vi "Follow Path Speed Control.vi"(0 "Drivetrain":T11={"DevStatus"={"status"=FALSE, "code"=0, "source"=""}, "Motors[]"=[{"DeviceStatus"={"status"=FALSE, "code"=0, "source"=""}, "Type"=enum."PWM", "PWM"={"PWM Channel"=enum."PWM 1", "DeadBand"={"Name"="SPARK", "maxPositivePwm"=1500, "minPositivePwm"=1010, "centerPwm"=1005, "maxNegativePwm"=1000, "minNegativePwm"=500, "angularRange"=0}}, "CAN"={"Device Number"=0, "SetOutput VI Ref"=variant(refnum<vi> refnum), "GetOutput VI Ref"=variant(refnum<vi> refnum), "Enable VI Ref"=variant(refnum<vi> refnum), "Disable VI Ref"=variant(refnum<vi> refnum), "Data"=variant}, "Invert"=TRUE}, {"DeviceStatus"={"status"=FALSE, "code"=0, "source"=""}, "Type"=enum."PWM", "PWM"={"PWM Channel"=enum."PWM 0", "DeadBand"={"Name"="SPARK", "maxPositivePwm"=1500, "minPositivePwm"=1010, "centerPwm"=1005, "maxNegativePwm"=1000, "minNegativePwm"=500, "angularRange"=0}}, "CAN"={"Device Number"=0, "SetOutput VI Ref"=variant(refnum<vi> refnum), "GetOutput VI Ref"=variant(refnum<vi> refnum), "Enable VI Ref"=variant(refnum<vi> refnum), "Disable VI Ref"=variant(refnum<vi> refnum), "Data"=variant}, "Invert"=FALSE}], "Square Inputs"=TRUE, "Max Output"=1.0}, 1 "Encoder L":T7={"DevStatus"={"status"=FALSE, "code"=0, "source"=""}, "EncoderIndex"=enum."Enc 0", "CounterIndex"=enum."Invalid", "DistancePerCount"=0.0490874, "Decoding Type"=enum."4x"}, 2 "Encoder R":T7={"DevStatus"={"status"=FALSE, "code"=0, "source"=""}, "EncoderIndex"=enum."Enc 1", "CounterIndex"=enum."Invalid", "DistancePerCount"=0.0490874, "Decoding Type"=enum."4x"}, 3 "Gyro":T4={"DevStatus"={"status"=FALSE, "code"=0, "source"=""}, "Analog Channel"=enum."AI 1", "Offset"=0.0, "Gain (VoltsPerDegree/Second)"=0.0, "Gyro Type"=enum."XRS450", "Handle"=27, "SPI Bus"=enum."SPI On-Board, CS0", "Device Found"=TRUE, "Sample Rate"=1.0, "Calibrate On Open"=FALSE} {"Sample Rate" min=0.25 max=100.0 step=0.25}, 4 "Trajectory":T2, 5 "error in":errorcluster, 6 "Queue in":refnum<queue>) -> (19 "error out":errorcluster)   [LabVIEW 2016, in "Drive System.lvlib"]
uses:
  Drive System.lvlib
  DriveCmd.ctl
  DriveCmdList.ctl
  <vilib>/Rock Robotics/WPI/RobotDrive/WPI_RobotDriveDevRef.ctl
  <vilib>/Rock Robotics/WPI/MotorControl/WPI_MotorControlDeviceRef.ctl
  <vilib>/Rock Robotics/WPI/MotorControl/WPI_MotorControlType.ctl
  <vilib>/Rock Robotics/SystemInterfaces/DIO/FPGA_DIOPWMChannel.ctl
  <vilib>/Rock Robotics/WPI/PWM/WPI_PWMDeadband.ctl
  <vilib>/Rock Robotics/WPI/Encoder/WPI_EncoderDevRef.ctl
  <vilib>/Rock Robotics/SystemInterfaces/Encoder/FPGA_EncoderIdx.ctl
  <vilib>/Rock Robotics/SystemInterfaces/Counter/FPGA_CounterCtrSystemIndex.ctl
  <vilib>/Rock Robotics/WPI/Encoder/WPI_EncoderType.ctl
  <vilib>/Rock Robotics/WPI/Gyro/WPI_GyroDevRef.ctl
  <vilib>/Rock Robotics/SystemInterfaces/AI/FPGA_AIChannel.ctl
  <vilib>/Rock Robotics/SystemInterfaces/spilib/spi_bus.ctl
  Varient Cmd Types/Follow Path.ctl
  Pathfinder/VIs/Segment.ctl
  <vilib>/Platform/TimedLoop/XDataNode/timing_clust.ctl
  <vilib>/Platform/TimedLoop/XDataNode/nitl_modes.ctl
  <vilib>/Platform/TimedLoop/XDataNode/wakeup.ctl
  Raw Data.vi
  <vilib>/Platform/TimedLoop/XDataNode/XDataNode.xnode
  <vilib>/Platform/TimedLoop/XDataNode/XDNodeRunTimeDep.lvlib
  <vilib>/ptbypt/NI_PtbyPt.lvlib
  Pathfinder/Pathfinder.lvlib
panel:
  out "Gyro":T1(graph)={"velocity"=-119.28017066681394, "output"=-0.08033081004418108, "mean"=-119.01240130000001}
  out "Waveform Chart 3":T1(graph)={"velocity"=-148.6015211300266, "output"=-0.12506612150797308, "mean"=-148.20713245000002}
  out "Waveform Chart 2":T1(graph)={"velocity"=-119.28017066681394, "output"=-0.08033081004418108, "mean"=-119.01240130000001}
  in  "Ka":dbl
  out "Waveform Chart":T1(graph)={"velocity"=-0.0, "output"=0.08512066021009909, "mean"=-1.2464638452949117}
  in  "Gains Position":cluster{"Kp":dbl, "Ki":dbl, "Kd":dbl, "Kf":dbl}={"Kp"=0.3, "Ki"=0.0, "Kd"=0.55, "Kf"=0.0} {"Kf" format="%.3f"; "Kd" format="%.3f"; "Ki" format="%.3f"; "Kp" format="%.3f"}
  in  "Gains Speed":cluster{"Kp":dbl, "Ki":dbl, "Kd":dbl, "Kf":dbl}={"Kp"=0.02, "Ki"=0.001, "Kd"=0.055, "Kf"=0.015} {"Kf" format="%.3f"; "Kd" format="%.3f"; "Ki" format="%.3f"; "Kp" format="%.3f"}
  in  "i Zone Speed":dbl=5.0 format="%.2f"
  in  "Output Range":cluster{"output high":dbl, "output low":dbl}={"output high"=1.0, "output low"=-1.0} {"output low" format="%.2f"; "output high" format="%.2f"}
  in  "Mean Samples":i32=32
  in  "Gains Gyro":cluster{"Kp":dbl, "Ki":dbl, "Kd":dbl, "Kf":dbl}={"Kp"=0.001, "Ki"=0.0, "Kd"=0.0, "Kf"=0.0} {"Kf" format="%.3f"; "Kd" format="%.3f"; "Ki" format="%.3f"; "Kp" format="%.3f"}
  in  "iZone":dbl=inf caption="iZone Gyro" format="%#_13g"
  in  "Gyro Invert":bool
  in  "Range":cluster{"output high":dbl, "output low":dbl}={"output high"=1.0, "output low"=-1.0} caption="Gyro output range" {"output low" format="%.2f"; "output high" format="%.2f"}
  # "Analog"
  # "XRS"
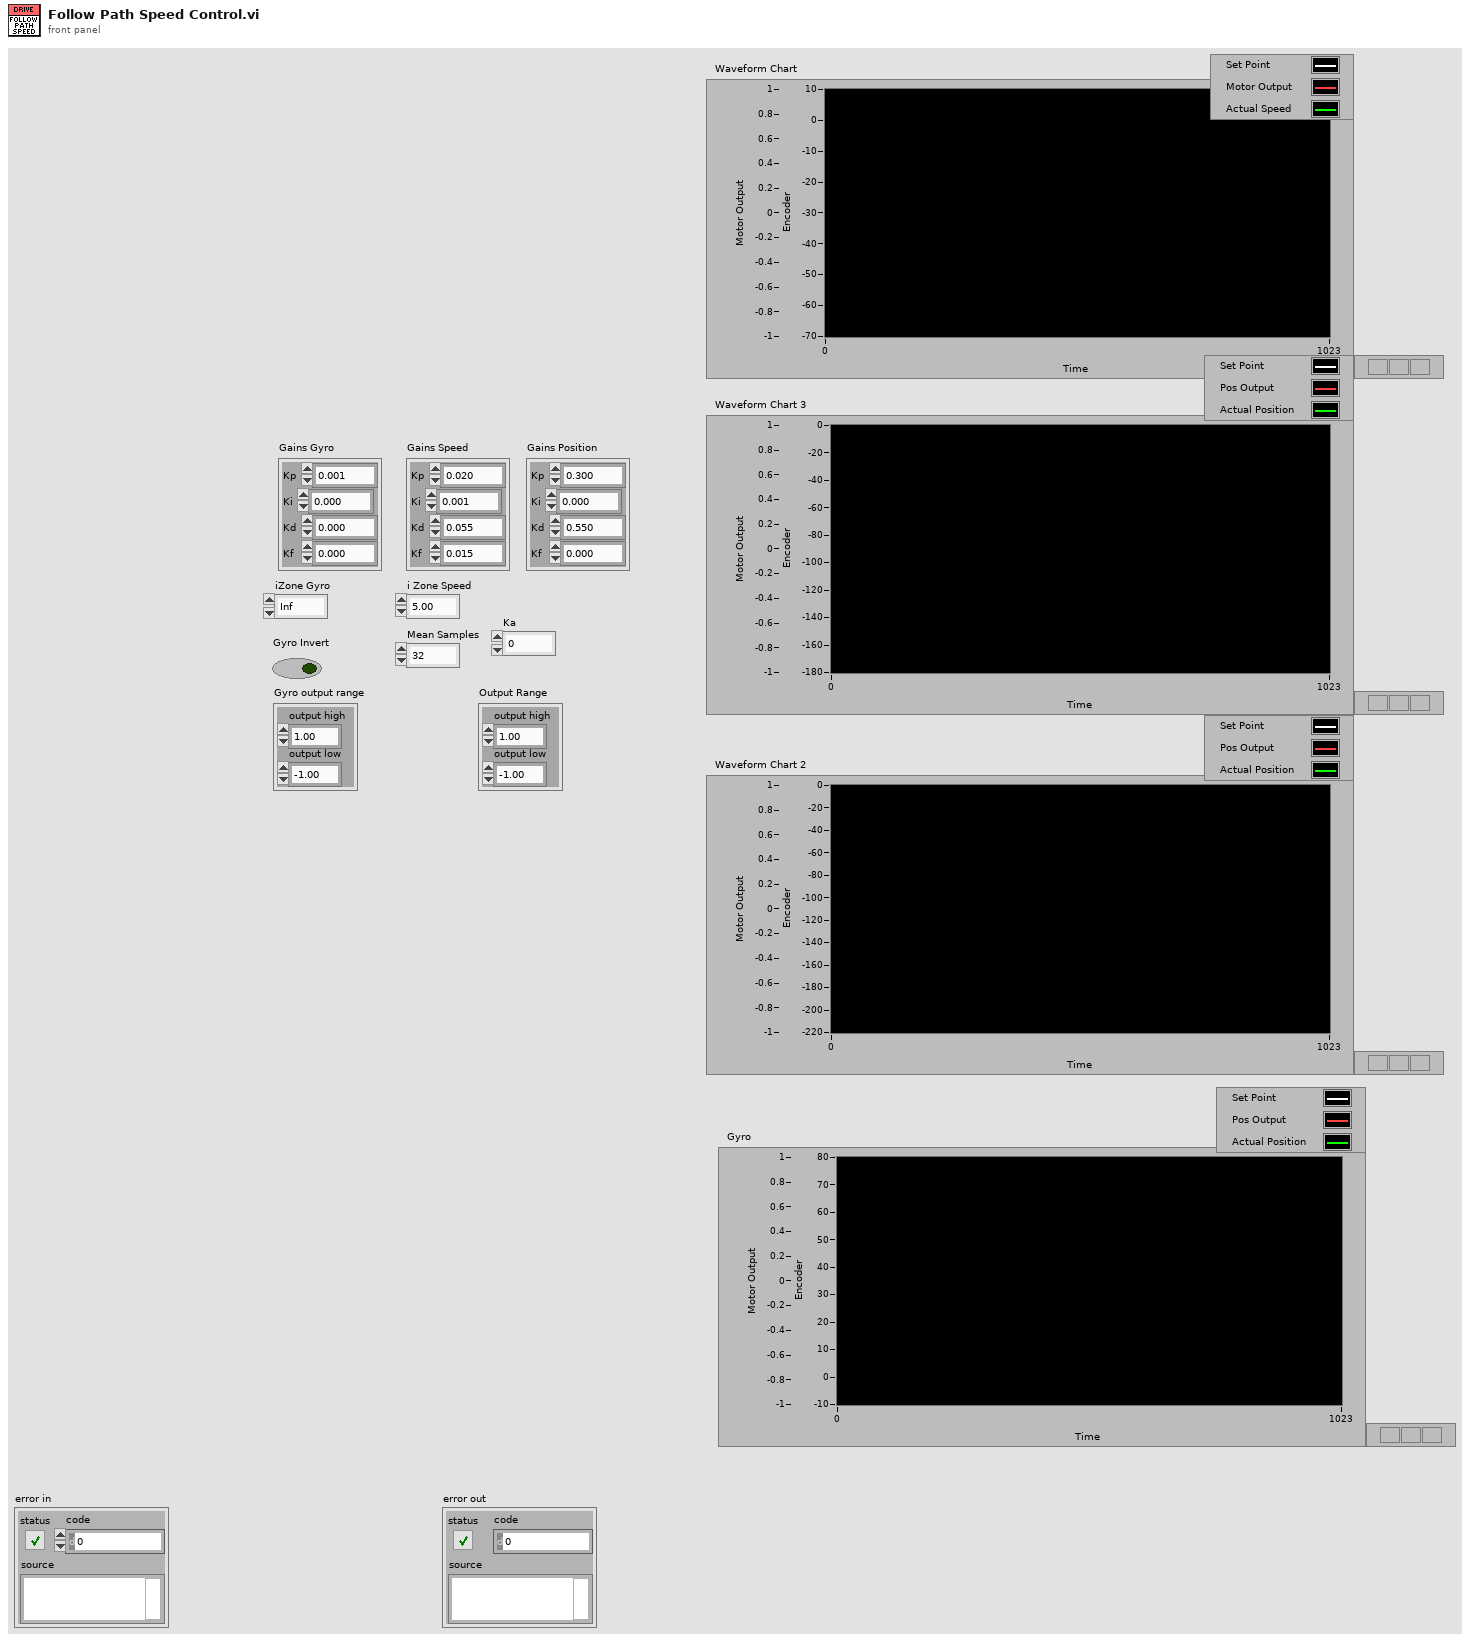
[diagram p1: front panel]
types:
  T1 = cluster{"velocity":dbl, "output":dbl, "mean":dbl}
  T2 = typedef "Drive System.lvlib/Follow Path.ctl" = cluster{"Left":T3[], "Right":T3[]}
  T3 = typedef "Pathfinder.lvlib/Segment.ctl" = cluster{"dt":dbl, "x":dbl, "y":dbl, "position":dbl, "velocity":dbl, "acceleration":dbl, "jerk":dbl, "heading":dbl}
  T4 = typedef "WPI_GyroDevRef.ctl" = cluster{"DevStatus":errorcluster, "Analog Channel":T5, "Offset":dbl, "Gain (VoltsPerDegree/Second)":dbl, "Gyro Type":enum16{"Analog", "XRS450"}, "Handle":i32, "SPI Bus":T6, "Device Found":bool, "Sample Rate":dbl, "Calibrate On Open":bool}
  T5 = typedef "FPGA_AIChannel.ctl" = enum8{"AI 0", "AI 1", "AI 2", "AI 3", "AI MXP 0", "AI MXP 1", "AI MXP 2", "AI MXP 3", "Invalid"}
  T6 = typedef "spi_bus.ctl" = enum16{"SPI On-Board, CS0", "SPI On-Board, CS1", "SPI On-Board, CS2", "SPI On-Board, CS3", "SPI MXP", "Invalid"}
  T7 = typedef "WPI_EncoderDevRef.ctl" = cluster{"DevStatus":errorcluster, "EncoderIndex":T8, "CounterIndex":T9, "DistancePerCount":dbl, "Decoding Type":T10}
  T8 = typedef "FPGA_EncoderIdx.ctl" = enum8{"Enc 0", "Enc 1", "Enc 2", "Enc 3", "Enc 4", "Enc 5", "Enc 6", "Enc 7", "Invalid"}
  T9 = typedef "FPGA_CounterCtrSystemIndex.ctl" = enum8{"Ctr 0", "Ctr 1", "Ctr 2", "Ctr 3", "Ctr 4", "Ctr 5", "Ctr 6", "Ctr 7", "Invalid"}
  T10 = typedef "WPI_EncoderType.ctl" = enum16{"1x", "2x", "4x"}
  T11 = typedef "WPI_RobotDriveDevRef.ctl" = cluster{"DevStatus":errorcluster, "Motors[]":T12[], "Square Inputs":bool, "Max Output":dbl}
  T12 = typedef "WPI_MotorControlDeviceRef.ctl" = cluster{"DeviceStatus":errorcluster, "Type":T13, "PWM":cluster{"PWM Channel":T14, "DeadBand":T15}, "CAN":cluster{"Device Number":u8, "SetOutput VI Ref":variant, "GetOutput VI Ref":variant, "Enable VI Ref":variant, "Disable VI Ref":variant, "Data":variant}, "Invert":bool}
  T13 = typedef "WPI_MotorControlType.ctl" = enum16{"PWM", "CAN"}
  T14 = typedef "FPGA_DIOPWMChannel.ctl" = enum8{"PWM 0", "PWM 1", "PWM 2", "PWM 3", "PWM 4", "PWM 5", "PWM 6", "PWM 7", "PWM 8", "PWM 9", "PWM MXP 0", "PWM MXP 1", "PWM MXP 2", "PWM MXP 3", "PWM MXP 4", "PWM MXP 5", "PWM MXP 6", "PWM MXP 7", "PWM MXP 8", "PWM MXP 9", "Invalid"}
  T15 = typedef "WPI_PWMDeadband.ctl" = cluster{"Name":string, "maxPositivePwm":i32, "minPositivePwm":i32, "centerPwm":i32, "maxNegativePwm":i32, "minNegativePwm":i32, "angularRange":u16}
  T16 = cluster{"Queue in":refnum<queue>, "Drivetrain":T11, "Encoder L":T7, "Encoder R":T7, "Gyro":T4}
  T17 = typedef "XDNodeRunTimeDep.lvlib/timing_clust.ctl" = cluster{"Expected End [f-1]":u64, "Actual End [f-1]":u64, "Finished Late? [f-1]":bool, "Expected End [i-1]":u64, "Actual End [i-1]":u64, "Finished Late? [i-1]":bool, "Expected Start [i]":u64, "Actual Start [i]":u64, "Expected Start [f]":u64, "Actual Start [f]":u64, "Source Name":string, "Structure Name":string, "Period":i64, "Deadline":i64, "Offset":i64, "Start":i64, "Priority":i32, "Timeout":i32, "Mode":T18, "Wakeup Reason":T19, "Error":errorcluster, "Source Type":string, "Secondary Source Type":string, "Global End Time":u64, "Global Start Time":u64, "Frame Duration":u64, "Iteration Duration":u64, "Assigned CPU":i32, "I/O Scan Engine Mode":u32}
  T18 = typedef "XDNodeRunTimeDep.lvlib/nitl_modes.ctl" = enum32{"No Change", "Process missed periods, maintain original phase", "Discard missed periods, maintain original phase", "Process missed periods, ignore original phase", "Discard missed periods, ignore original phase"}
  T19 = typedef "XDNodeRunTimeDep.lvlib/wakeup.ctl" = enum32{"Normal", "Aborted", "Asynchronous wakeup", "Timing source error", "Timed loop error", "Timeout"}
  T20 = cluster{"position":dbl, "position output":dbl, "Distance":dbl}
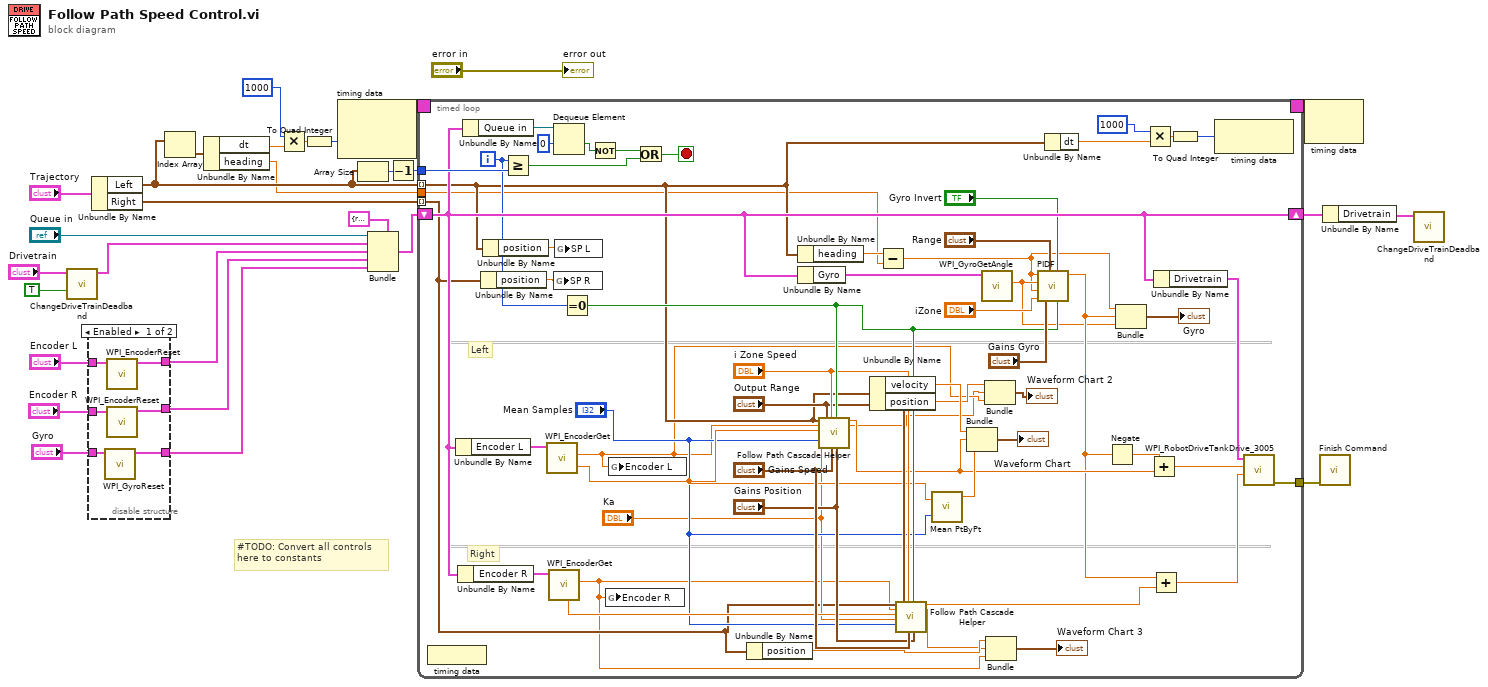
[diagram p0: block diagram]
diagram:
  # "#TODO: Convert all controls\nhere to constants"
  n1 = call "ChangeDriveTrainDeadband.vi"("Eliminate Deadband"=TRUE, "Drivetrain in"="Drivetrain") -> ("Drivetrain out"=w13:T11)  [unwired: 9 in]
  n2 = disable-structure shown="Enabled" {
    disable-tunnel: "Encoder R" -> [w35 _]
    disable-tunnel: "Encoder L" -> [w34 _]
    disable-tunnel: "Gyro" -> [w33 _]
    disable-tunnel: [w32 _] -> w6
    disable-tunnel: [w31 _] -> w5
    disable-tunnel: [w30 _] -> w4
    frame Enabled {
      n3 = call <vilib>:"WPI_GyroReset.vi"("GyroDevRef"=w33) -> ("GyroDevRef"=w30:T4)  [unwired: 9 in, 1 out]
      n4 = call <vilib>:"WPI_EncoderReset.vi"("EncoderDevRef"=w34) -> ("EncoderDevRef"=w32:T7)  [unwired: 9 in, 1 out]
      n5 = call <vilib>:"WPI_EncoderReset.vi"("EncoderDevRef"=w35) -> ("EncoderDevRef"=w31:T7)  [unwired: 9 in, 1 out]
    }
    frame Disabled {
    }
  }
  n6 = Unbundle By Name("Trajectory") -> ("Left"=w18:T3[], "Right"=w19:T3[])
  n7 = Index Array(array=w18) -> (element=w25:T3)  [unwired: 1 in]
  n8 = Unbundle By Name(w25) -> ("dt"=w2:dbl, "heading"=w1:dbl)
  n9 = Multiply(x=i64 1000 ("Period"), y=w2) -> (x*y=w22:dbl)
  n10 = To Quad Integer(1:w22) -> (0:w23:i64)
  n11 = node-c288(w23) -> (w29:T17)  [unwired: 1 in]
  n12 = Array Size(array=w18) -> (size(s)=w17:i32)
  n13 = Bundle(cluster=T16 {"Queue in"=refnum, "Drivetrain"={"DevStatus"={"status"=FALSE, "code"=0, "source"=""}, "Motors[]"=[], "Square Inputs"=FALSE, "Max Output"=0.0}, "Encoder L"={"DevStatus"={"status"=FALSE, "code"=0, "source"=""}, "EncoderIndex"=enum."Enc 0", "CounterIndex"=enum."Ctr 0", "DistancePerCount"=0.0, "Decoding Type"=enum."1x"}, "Encoder R"={"DevStatus"={"status"=FALSE, "code"=0, "source"=""}, "EncoderIndex"=enum."Enc 0", "CounterIndex"=enum."Ctr 0", "DistancePerCount"=0.0, "Decoding Type"=enum."1x"}, "Gyro"={"DevStatus"={"status"=FALSE, "code"=0, "source"=""}, "Analog Channel"=enum."AI 0", "Offset"=0.0, "Gain (VoltsPerDegree/Second)"=0.0, "Gyro Type"=enum."Analog", "Handle"=0, "SPI Bus"=enum."SPI On-Board, CS0", "Device Found"=FALSE, "Sample Rate"=0.0, "Calibrate On Open"=FALSE}}, "Queue in"="Queue in", "Drivetrain"=w13, "Encoder L"=w6, "Encoder R"=w5, "Gyro"=w4) -> (w21:T16)
  n14 = Decrement(x=w17) -> (x-1=w16:i32)
  n15 = timed-loop {
    timing: w29 -> [_]
    timing-out: [_] -> w28
    shift-right: [w79] -> w11
    shift-left: w21 -> [w79]
    tunnel: w19 -> [w46] mode=indexing
    tunnel: w18 -> [w54] mode=indexing
    tunnel: w16 -> [w85]
    tunnel: [w69] -> w15
    tunnel: w1 -> [w36]
    i -> [w67]
    stop <- w87 stop-if-true
    # "Left"
    # "Right"
    n16 = node-c288() -> ()  [unwired: 1 in]
    n17 = Unbundle By Name(w79) -> ("Encoder L"=w82:T7)
    n18 = Unbundle By Name(w79) -> ("Encoder R"=w81:T7)
    n19 = Unbundle By Name(w79) -> ("Queue in"=w90:refnum<queue>)
    n20 = Unbundle By Name(w46) -> ("position"=w74:dbl)
    n21 = Unbundle By Name(w54) -> ("position"=w75:dbl)
    n22 = Greater Or Equal?(x=w67, y=w85) -> (x >= y?=w84:bool)
    n23 = call <vilib>:"WPI_EncoderGet.vi"("EncoderDevRef"=w82) -> ("Distance"=w49:dbl, "Rate"=w58:dbl)  [unwired: 5 in, 4 out]
    n24 = call <vilib>:"WPI_EncoderGet.vi"("EncoderDevRef"=w81) -> ("Distance"=w43:dbl, "Rate"=w60:dbl)  [unwired: 5 in, 4 out]
    n25 = Dequeue Element(queue=w90, timeout in ms (-1)=0) -> (timed out?=w68:bool)  [unwired: 1 in, 3 out]
    n26 = global write "Raw Data.vi" "SP R"(w74) -> ()
    n27 = global write "Raw Data.vi" "SP L"(w75) -> ()
    n28 = Equal To 0?(x=w67) -> (x = 0?=w66:bool)
    n29 = Not(x=w68) -> (.not. x?=w86:bool)
    n30 = global write "Raw Data.vi" "Encoder R"(w43) -> ()
    n31 = global write "Raw Data.vi" "Encoder L"(w49) -> ()
    n32 = Or(x=w86, y=w84) -> (x .or. y?=w87:bool)
    n33 = Unbundle By Name(w46) -> ("position"=w45:dbl)
    n34 = Unbundle By Name(w54) -> ("heading"=w38:dbl)
    n35 = Unbundle By Name(w79) -> ("Gyro"=w78:T4)
    n36 = call "Follow Path Cascade Helper.vi"("segment"=w54, "Encoder Position"=w49, "Encoder Rate"=w58, "Ka"="Ka", "Encoder Mean Samples"="Mean Samples", "Output Range"="Output Range", "i Zone Speed"="i Zone Speed", "Gains Speed"="Gains Speed", "Reinitialize"=w66, "Gains Position"="Gains Position") -> ("output"=w50:dbl, "position output"=w47:dbl)  [unwired: 8 in]
    n37 = Unbundle By Name(w54) -> ("velocity"=w53:dbl, "position"=w51:dbl)
    n38 = Subtract(x=w38, y=w36) -> (x-y=w37:dbl)
    n39 = call "Follow Path Cascade Helper.vi"("segment"=w46, "Encoder Position"=w43, "Encoder Rate"=w60, "Ka"="Ka", "Encoder Mean Samples"="Mean Samples", "Output Range"="Output Range", "i Zone Speed"="i Zone Speed", "Gains Speed"="Gains Speed", "Reinitialize"=w66, "Gains Position"="Gains Position") -> ("output"=w63:dbl, "position output"=w44:dbl)  [unwired: 8 in]
    n40 = call <vilib>:"Mean PtByPt.vi"("x"=w58, "sample length"="Mean Samples") -> ("mean"=w56:dbl)  [unwired: 2 in, 1 out]
    n41 = Bundle("velocity"=w53, "output"=w50, "mean"=w56) -> (→"Waveform Chart":T1)  [unwired: 1 in]
    n42 = call <vilib>:"WPI_GyroGetAngle.vi"("GyroDevRef"=w78) -> ("Angle"=w40:dbl)  [unwired: 6 in, 4 out]
    n43 = Bundle("position"=w51, "position output"=w47, "Distance"=w49) -> (→"Waveform Chart 2":T20)  [unwired: 1 in]
    n44 = Bundle("position"=w45, "position output"=w44, "Distance"=w43) -> (→"Waveform Chart 3":T20)  [unwired: 1 in]
    n45 = call "PIDF.vi"("reinitialize? (F)"=w66, "invert? (F)"="Gyro Invert", "PIDF gains"="Gains Gyro", "output range"="Range", "i Zone"="iZone", "Feedforward"=w37, "process variable"=w40, "setpoint"=w37) -> ("output"=w41:dbl)  [unwired: 1 in, 2 out]
    n46 = Unbundle By Name(w54) -> ("dt"=w83:dbl)
    n47 = Negate(x=w41) -> (-x=w55:dbl)
    n48 = Bundle(w37, "output"=w41, "Angle"=w40) -> (→"Gyro":cluster{dbl, "output":dbl, "Angle":dbl})  [unwired: 1 in]
    n49 = Multiply(x=i64 1000 ("Period"), y=w83) -> (x*y=w92:dbl)
    n50 = Add(x=w55, y=w50) -> (x+y=w77:dbl)
    n51 = Add(x=w41, y=w63) -> (x+y=w76:dbl)
    n52 = Unbundle By Name(w79) -> ("Drivetrain"=w80:T11)
    n53 = To Quad Integer(1:w92) -> (0:w91:i64)
    n54 = node-c288(w91) -> ()  [unwired: 1 out]
    n55 = call "WPI_RobotDriveTankDrive_3005.vi"("Right axis value"=w76, "Left axis value"=w77, "RobotDriveDevRef"=w80) -> ("error out"=w69:errorcluster)  [unwired: 7 in, 1 out]
  }
  n56 = node-c288(w28) -> ()  [unwired: 1 out]
  n57 = call "Finish Command.vi"("error in"=w15) -> ()  [unwired: 10 in, 1 out]
  n58 = Unbundle By Name(w11) -> ("Drivetrain"=w10:T11)
  n59 = call "ChangeDriveTrainDeadband.vi"("Drivetrain in"=w10) -> ()  [unwired: 10 in, 1 out]
  "error out" <- "error in"
